vi "Lockin Read Data.vi"(7 "DAQ timeout, s":dbl=10.0 format="%0.2f", 8 "error in (no error)":errorcluster, 10 "DAQ task":refnum<k21>, 11 "Lock-in settings":T1={"Sine Frequency, Hz"=0.0, "Time constant, s"=0.12500000000000006, "Low-pass filter"=enum."No filtering", "Output representation"=enum."Real/Imaginary", "Phases, deg"=[], "Low-pass filter Order"=1, "Decimating factor"=1, "Samples to Read"=10000, "Post-filter decimation"=1, "Blocks to average"=1, "Trig delay, points"=0, "Harmonics per channel"=[], "Amplitude scale"=enum."RMS"} {"Time constant, s" format="%.1e"}) -> (0 "error out":errorcluster, 2 "task out":refnum<k21>, 3 "Lock-in settings out":T1={"Sine Frequency, Hz"=0.0, "Time constant, s"=0.12500000000000006, "Low-pass filter"=enum."No filtering", "Output representation"=enum."Real/Imaginary", "Phases, deg"=[], "Low-pass filter Order"=1, "Decimating factor"=1, "Samples to Read"=10000, "Post-filter decimation"=1, "Blocks to average"=1, "Trig delay, points"=0, "Harmonics per channel"=[], "Amplitude scale"=enum."RMS"} {"Time constant, s" format="%.1e"}, 4 "AvailSampPerChan":u32, 5 "data":waveform(dbl)[](array[waveform]))   [LabVIEW 2020]
uses:
  Lockin Settings.ctl
  Harmonics per channel.ctl
  <vilib>/DAQmx/read.llb/DAQmx Read (Analog 1D Wfm NChan NSamp).vi
  <vilib>/DAQmx/miscellaneous.llb/DAQmx Fill In Error Info.vi
  <resource>/objmgr/daqmx.rc
panel:
  out "SampClk.Src":tag
  out "SampClk.Rate":dbl
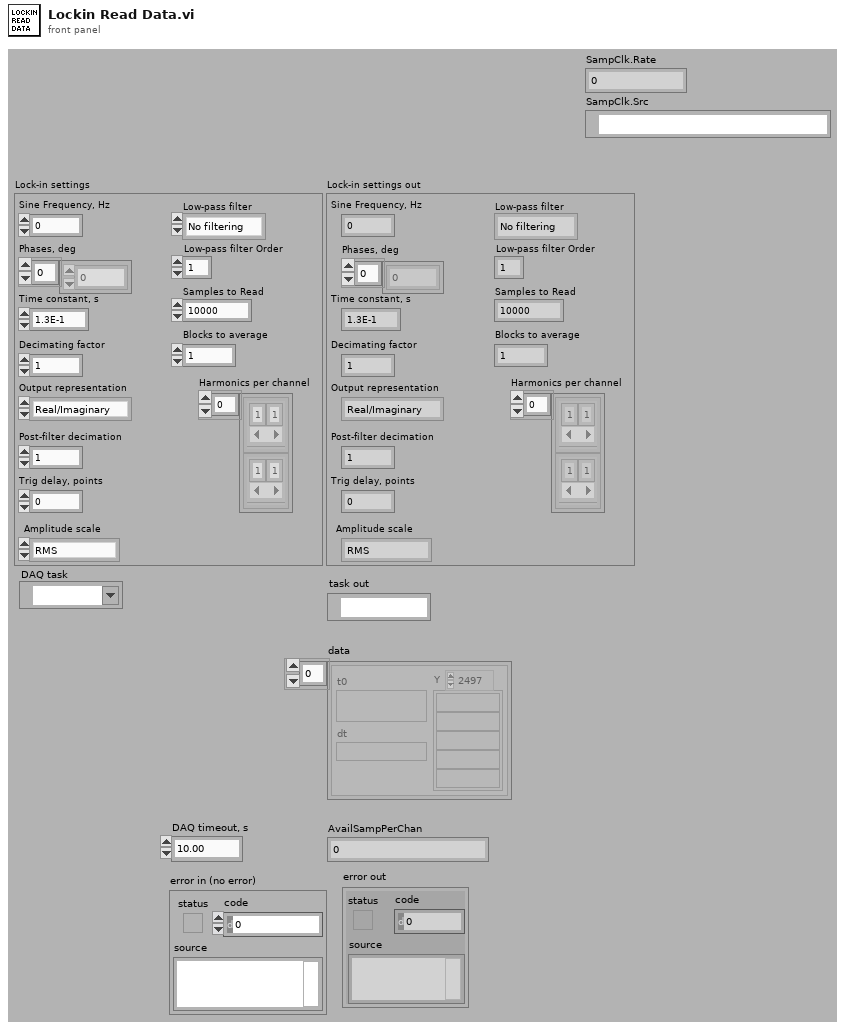
[diagram p1: front panel]
types:
  T1 = typedef "Lockin Settings.ctl" = cluster{"Sine Frequency, Hz":dbl, "Time constant, s":dbl, "Low-pass filter":enum16{"No filtering", "Butterworth", "Bessel"}, "Output representation":enum16{"Real/Imaginary", "Polar"}, "Phases, deg":dbl[], "Low-pass filter Order":i32, "Decimating factor":i32, "Samples to Read":i32, "Post-filter decimation":i32, "Blocks to average":i32, "Trig delay, points":i32, "Harmonics per channel":T2, "Amplitude scale":enum16{"Amplitude", "RMS", "Peak-to-Peak"}}
  T2 = typedef "Harmonics per channel.ctl" = cluster{"Harmonics":i32[]}[]
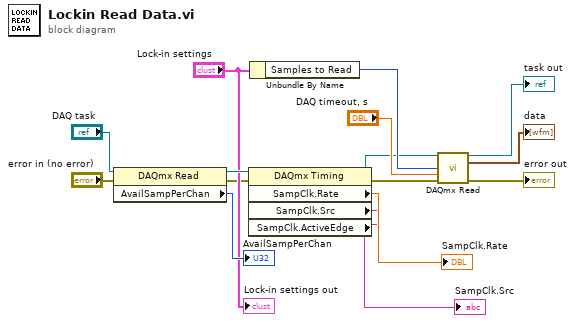
[diagram p0: block diagram]
diagram:
  n1 = property class="DAQmx Read"(reference="DAQ task", error in="error in (no error)") -> (reference out=w12:refnum<k21>, error out=w4:errorcluster, "AvailSampPerChan"=→"AvailSampPerChan":u32)
  n2 = property class="DAQmx Timing" props=["SampClk.Rate", "SampClk.Src", "SampClk.ActiveEdge"](reference=w12, error in=w4) -> (reference out=w5:refnum<k21>, error out=w3:errorcluster, "SampClk.Rate"=→"SampClk.Rate":dbl, "SampClk.Src"=→"SampClk.Src":tag)  [unwired: 1 out]
  n3 = Unbundle By Name("Lock-in settings") -> ("Samples to Read"=w14:i32)
  n4 = call-poly <vilib>:"DAQmx Read.vi"("task/channels in"=w5, "number of samples per channel"=w14, "timeout"="DAQ timeout, s", "error in"=w3) -> ("task out"=→"task out":refnum<k21>, "data"=→"data":waveform(dbl)[], "error out"=→"error out":errorcluster)  [unwired: 9 out]
  "Lock-in settings out" <- "Lock-in settings"
